vi "format_heading.vi"(1 "Heading (deg)":i32(knob) scale=-360.0..360.0) -> (0 "heading (formatted)":T1)   [LabVIEW 2015]
uses:
  <vilib>/express/express arith-compare/Formula/XNode/ExpressFormulaBlockNode.xnode
panel:
  in  "Circle init":dbl[][](array[numeric])=[[15.0, 30.0], [16.30733614, 29.94292047], [17.60472267, 29.7721163], [17.43107449, 28.78730854], [17.60472267, 29.7721163], [18.88228568, 29.48888739], [20.13030215, 29.09538931], [19.78828201, 28.15569669], [20.13030215, 29.09538931], [21.33927393, 28.59461681], [22.5, 27.99038106], [22.0, 27.12435565], [22.5, 27.99038106], [23.60364655, 27.28728066], [24.64181415, 26.49066665], [23.99902654, 25.7246222], [24.64181415, 26.49066665], [25.60660172, 25.60660172], [26.49066665, 24.64181415], [25.7246222, 23.99902654], [26.49066665, 24.64181415], [27.28728066, 23.60364655], [27.99038106, 22.5], [27.12435565, 22.0], [27.99038106, 22.5], [28.59461681, 21.33927393], [29.09538931, 20.13030215], [28.15569669, 19.78828201], [29.09538931, 20.13030215], [29.48888739, 18.88228568], [29.7721163, 17.60472267], [28.78730854, 17.43107449], [29.7721163, 17.60472267], [29.94292047, 16.30733614], [30.0, 15.0], [28.5, 15.0], [30.0, 15.0], [29.94292047, 13.69266386], [29.7721163, 12.39527733], [28.78730854, 12.56892551], [29.7721163, 12.39527733], [29.48888739, 11.11771432], [29.09538931, 9.86969785], [28.15569669, 10.21171799], [29.09538931, 9.86969785], [28.59461681, 8.660726074], [27.99038106, 7.5], [27.12435565, 8.0], [27.99038106, 7.5], [27.28728066, 6.396353455], [26.49066665, 5.358185855], [25.7246222, 6.000973464], [26.49066665, 5.358185855], [25.60660172, 4.393398282], [24.64181415, 3.509333353], [23.99902654, 4.275377796], [24.64181415, 3.509333353], [23.60364655, 2.712719336], [22.5, 2.009618943], [22.0, 2.875644347], [22.5, 2.009618943], [21.33927393, 1.405383194], [20.13030215, 0.904610688], [19.78828201, 1.844303309], [20.13030215, 0.904610688], [18.88228568, 0.511112606], [17.60472267, 0.227883705], [17.43107449, 1.212691458], [17.60472267, 0.227883705], [16.30733614, 0.057079529], [15.0, 0.0], [15.0, 1.5], [15.0, 0.0], [13.69266386, 0.057079529], [12.39527733, 0.227883705], [12.56892551, 1.212691458], [12.39527733, 0.227883705], [11.11771432, 0.511112606], [9.86969785, 0.904610688], [10.21171799, 1.844303309], [9.86969785, 0.904610688], [8.660726074, 1.405383194], [7.5, 2.009618943], [8.0, 2.875644347], [7.5, 2.009618943], [6.396353455, 2.712719336], [5.358185855, 3.509333353], [6.000973464, 4.275377796], [5.358185855, 3.509333353], [4.393398282, 4.393398282], [3.509333353, 5.358185855], [4.275377796, 6.000973464], [3.509333353, 5.358185855], [2.712719336, 6.396353455], [2.009618943, 7.5], [2.875644347, 8.0], [2.009618943, 7.5], [1.405383194, 8.660726074], [0.904610688, 9.86969785], [1.844303309, 10.21171799], [0.904610688, 9.86969785], [0.511112606, 11.11771432], [0.227883705, 12.39527733], [1.212691458, 12.56892551], [0.227883705, 12.39527733], [0.057079529, 13.69266386], [0.0, 15.0], [1.5, 15.0], [0.0, 15.0], [0.057079529, 16.30733614], [0.227883705, 17.60472267], [1.212691458, 17.43107449], [0.227883705, 17.60472267], [0.511112606, 18.88228568], [0.904610688, 20.13030215], [1.844303309, 19.78828201], [0.904610688, 20.13030215], [1.405383194, 21.33927393], [2.009618943, 22.5], [2.875644347, 22.0], [2.009618943, 22.5], [2.712719336, 23.60364655], [3.509333353, 24.64181415], [4.275377796, 23.99902654], [3.509333353, 24.64181415], [4.393398282, 25.60660172], [5.358185855, 26.49066665], [6.000973464, 25.7246222], [5.358185855, 26.49066665], [6.396353455, 27.28728066], [7.5, 27.99038106], [8.0, 27.12435565], [7.5, 27.99038106], [8.660726074, 28.59461681], [9.86969785, 29.09538931], [10.21171799, 28.15569669], [9.86969785, 29.09538931], [11.11771432, 29.48888739], [12.39527733, 29.7721163], [12.56892551, 28.78730854], [12.39527733, 29.7721163], [13.69266386, 29.94292047], [15.0, 30.0], [15.0, 28.5]] format="%0.3f"
  in  "Aircraft init":dbl[][](array[numeric])=[[10.30776406, 165.9637565], [11.18033989, 153.4349488], [5.024937811, 95.71059314], [12.0, 90.0], [5.024937811, 84.28940686], [11.18033989, 26.56505118], [10.30776406, 14.03624347], [2.549509757, 78.69006753], [7.516648189, -86.18592517], [10.29563014, -60.9453959], [11.18033989, -63.43494882], [11.18033989, -116.5650512], [10.29563014, -119.0546041], [7.516648189, -93.81407483], [2.549509757, 101.3099325], [10.30776406, 165.9637565]] format="%0.3f"
  out "Aircraft":cluster{"Y":dbl[], "Y":dbl[]}[](array[cluster])
  out "Circle":cluster{"Y":dbl[], "Y":dbl[]}[](array[cluster])
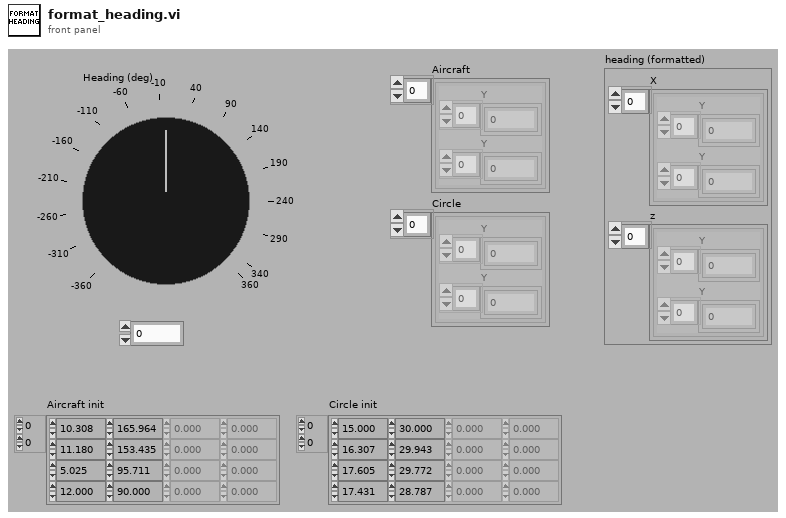
[diagram p1: front panel]
types:
  T1 = cluster{"X":cluster{"Y":dbl[], "Y":dbl[]}[], "z":cluster{"Y":dbl[], "Y":dbl[]}[]}
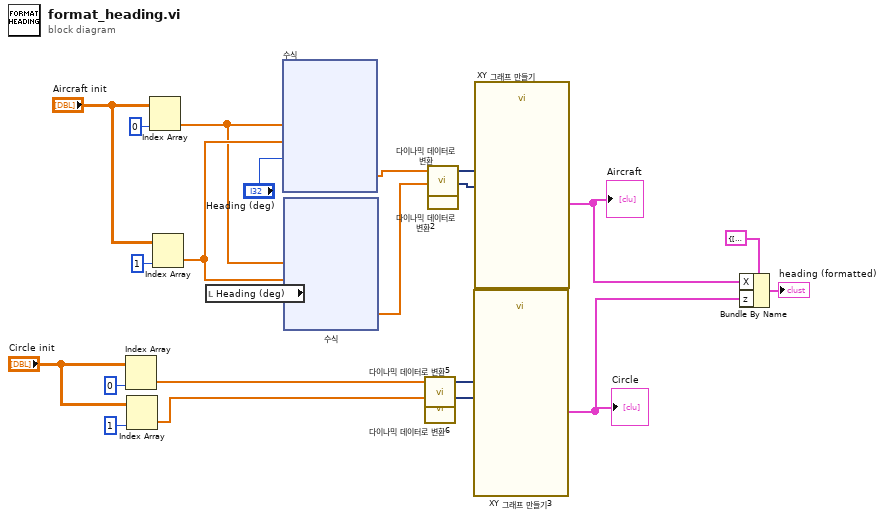
[diagram p0: block diagram]
diagram:
  n1 = Index Array(array="Circle init", index (col)=0 ("인덱스 (행)")) -> (element=w17:dbl[])  [unwired: 1 in]
  n2 = Index Array(array="Circle init", index (col)=1 ("비활성화된 인덱스 (열)")) -> (element=w19:dbl[])  [unwired: 1 in]
  n3 = Index Array(array="Aircraft init", index (col)=0 ("인덱스 (행)")) -> (element=w13:dbl[])  [unwired: 1 in]
  n4 = Index Array(array="Aircraft init", index (col)=1 ("비활성화된 인덱스 (열)")) -> (element=w14:dbl[])  [unwired: 1 in]
  n5 = local read "Heading (deg)"() -> (w5:i32)
  n6 = xnode "수식"("X1"=w13, "X2"=w14, "X3"="Heading (deg)") -> ("결과"=w11:dbl[])  [unwired: 1 in, 1 out]
  n7 = xnode "수식"("X1"=w13, "X2"=w14, "X3"=w5) -> ("결과"=w12:dbl[])  [unwired: 1 in, 1 out]
  n8 = call "다이나믹 데이터로 변환5"("Array"=w17) -> ("Dynamic Data Type"=w18:dynamicdata)  [unwired: 3 in]
  n9 = call "다이나믹 데이터로 변환6"("Array"=w19) -> ("Dynamic Data Type"=w20:dynamicdata)  [unwired: 3 in]
  n10 = call "다이나믹 데이터로 변환"("Array"=w11) -> ("Dynamic Data Type"=w8:dynamicdata)  [unwired: 3 in]
  n11 = call "다이나믹 데이터로 변환2"("Array"=w12) -> ("Dynamic Data Type"=w9:dynamicdata)  [unwired: 3 in]
  n12 = call "XY 그래프 만들기3"("Y Input"=w20, "X Input"=w18) -> ("XY Graph"=w2:cluster{"Y":dbl[], "Y":dbl[]}[])  [unwired: 8 in, 1 out]
  "Circle" <- w2
  n13 = call "XY 그래프 만들기"("Y Input"=w9, "X Input"=w8) -> ("XY Graph"=w3:cluster{"Y":dbl[], "Y":dbl[]}[])  [unwired: 8 in, 1 out]
  "Aircraft" <- w3
  n14 = Bundle By Name(cluster=T1 {"X"=[{"Y"=[21.620706805998168, 20.15124367946963, 12.465582235692763, 7.946576972490323, 11.656565240893995, 3.970903792227472, 5.440366929130449, 13.126028372052978, 19.003880895383112, 16.244982298473555, 16.832767550897515, 24.922937499080067, 24.33515224168201, 19.81289788882929, 13.93504536742159, 21.620706805998168], "Y"=[7.099604990531346, 5.077062500919932, 10.661022401488875, 5.291796067500631, 11.248807654089271, 16.832767550897515, 18.855310035128806, 13.271350139939326, 21.36152008350073, 25.220079209877188, 26.02909620777253, 20.151243679469633, 19.34222668734553, 20.773734831883043, 12.683564887248515, 7.099604990531346]}], "z"=[{"Y"=[15.0, 16.30733614, 17.60472267, 17.43107449, 17.60472267, 18.88228568, 20.13030215, 19.78828201, 20.13030215, 21.33927393, 22.5, 22.0, 22.5, 23.60364655, 24.64181415, 23.99902654, 24.64181415, 25.60660172, 26.49066665, 25.7246222, 26.49066665, 27.28728066, 27.99038106, 27.12435565, 27.99038106, 28.59461681, 29.09538931, 28.15569669, 29.09538931, 29.48888739, 29.7721163, 28.78730854, 29.7721163, 29.94292047, 30.0, 28.5, 30.0, 29.94292047, 29.7721163, 28.78730854, 29.7721163, 29.48888739, 29.09538931, 28.15569669, 29.09538931, 28.59461681, 27.99038106, 27.12435565, 27.99038106, 27.28728066, 26.49066665, 25.7246222, 26.49066665, 25.60660172, 24.64181415, 23.99902654, 24.64181415, 23.60364655, 22.5, 22.0, 22.5, 21.33927393, 20.13030215, 19.78828201, 20.13030215, 18.88228568, 17.60472267, 17.43107449, 17.60472267, 16.30733614, 15.0, 15.0, 15.0, 13.69266386, 12.39527733, 12.56892551, 12.39527733, 11.11771432, 9.86969785, 10.21171799, 9.86969785, 8.660726074, 7.5, 8.0, 7.5, 6.396353455, 5.358185855, 6.000973464, 5.358185855, 4.393398282, 3.509333353, 4.275377796, 3.509333353, 2.712719336, 2.009618943, 2.875644347, 2.009618943, 1.405383194, 0.904610688, 1.844303309, 0.904610688, 0.511112606, 0.227883705, 1.212691458, 0.227883705, 0.057079529, 0.0, 1.5, 0.0, 0.057079529, 0.227883705, 1.212691458, 0.227883705, 0.511112606, 0.904610688, 1.844303309, 0.904610688, 1.405383194, 2.009618943, 2.875644347, 2.009618943, 2.712719336, 3.509333353, 4.275377796, 3.509333353, 4.393398282, 5.358185855, 6.000973464, 5.358185855, 6.396353455, 7.5, 8.0, 7.5, 8.660726074, 9.86969785, 10.21171799, 9.86969785, 11.11771432, 12.39527733, 12.56892551, 12.39527733, 13.69266386, 15.0, 15.0], "Y"=[30.0, 29.94292047, 29.7721163, 28.78730854, 29.7721163, 29.48888739, 29.09538931, 28.15569669, 29.09538931, 28.59461681, 27.99038106, 27.12435565, 27.99038106, 27.28728066, 26.49066665, 25.7246222, 26.49066665, 25.60660172, 24.64181415, 23.99902654, 24.64181415, 23.60364655, 22.5, 22.0, 22.5, 21.33927393, 20.13030215, 19.78828201, 20.13030215, 18.88228568, 17.60472267, 17.43107449, 17.60472267, 16.30733614, 15.0, 15.0, 15.0, 13.69266386, 12.39527733, 12.56892551, 12.39527733, 11.11771432, 9.86969785, 10.21171799, 9.86969785, 8.660726074, 7.5, 8.0, 7.5, 6.396353455, 5.358185855, 6.000973464, 5.358185855, 4.393398282, 3.509333353, 4.275377796, 3.509333353, 2.712719336, 2.009618943, 2.875644347, 2.009618943, 1.405383194, 0.904610688, 1.844303309, 0.904610688, 0.511112606, 0.227883705, 1.212691458, 0.227883705, 0.057079529, 0.0, 1.5, 0.0, 0.057079529, 0.227883705, 1.212691458, 0.227883705, 0.511112606, 0.904610688, 1.844303309, 0.904610688, 1.405383194, 2.009618943, 2.875644347, 2.009618943, 2.712719336, 3.509333353, 4.275377796, 3.509333353, 4.393398282, 5.358185855, 6.000973464, 5.358185855, 6.396353455, 7.5, 8.0, 7.5, 8.660726074, 9.86969785, 10.21171799, 9.86969785, 11.11771432, 12.39527733, 12.56892551, 12.39527733, 13.69266386, 15.0, 15.0, 15.0, 16.30733614, 17.60472267, 17.43107449, 17.60472267, 18.88228568, 20.13030215, 19.78828201, 20.13030215, 21.33927393, 22.5, 22.0, 22.5, 23.60364655, 24.64181415, 23.99902654, 24.64181415, 25.60660172, 26.49066665, 25.7246222, 26.49066665, 27.28728066, 27.99038106, 27.12435565, 27.99038106, 28.59461681, 29.09538931, 28.15569669, 29.09538931, 29.48888739, 29.7721163, 28.78730854, 29.7721163, 29.94292047, 30.0, 28.5]}]} ("Heading"), "X"=w3, "z"=w2) -> (→"heading (formatted)":T1)
